vi "Pulse Measurements 1 chan (obs).vi"(6 "percent level settings":T2={"method"=enum."auto select", "histogram size"=256, "histogram method"=enum."mode", "reserved"=1.0} {"reserved" format="%0.2f"}, 7 "pulse number (1)":i32=1 min=1, 8 "error in (no error)":errorcluster, 9 "reference levels":T3={"high ref level"=90.0, "mid ref level"=50.0, "low ref level"=10.0, "ref units"=1} {"ref units" items=["absolute", "percent"]; "high ref level" format="%0.2f"; "low ref level" format="%0.2f"; "mid ref level" format="%0.2f"}, 10 "polarity (high)":u16(ring)=1 items=["low pulse", "high pulse"], 11 "signal in":waveform(dbl)={"t0"=timestamp(0 s since 1904-01-01), "dt"=0.0, "Y"=[]}) -> (0 "error out":errorcluster, 1 "duty cycle":dbl format="%.2g", 2 "pulse duration":dbl format="%.2g", 3 "period":dbl format="%.2g", 4 "measurement info":T1 {"ref levels"."ref units" items=["absolute", "relative"]; "ref levels"."high ref level" format="%.2p"; "ref levels"."low ref level" format="%.2p"; "ref levels"."mid ref level" format="%.2p"; "pulse center" format="%.2p"})   [LabVIEW 2020, in "NI_MAPro.lvlib"]
uses:
  NI_MAPro.lvlib
  <resource>/lvanlys.dll
  NI_MABase.lvlib
panel:
  # "This VI is obsolete !!!\nYou should replace this VI in your diagram with the Pulse Measurements VI."
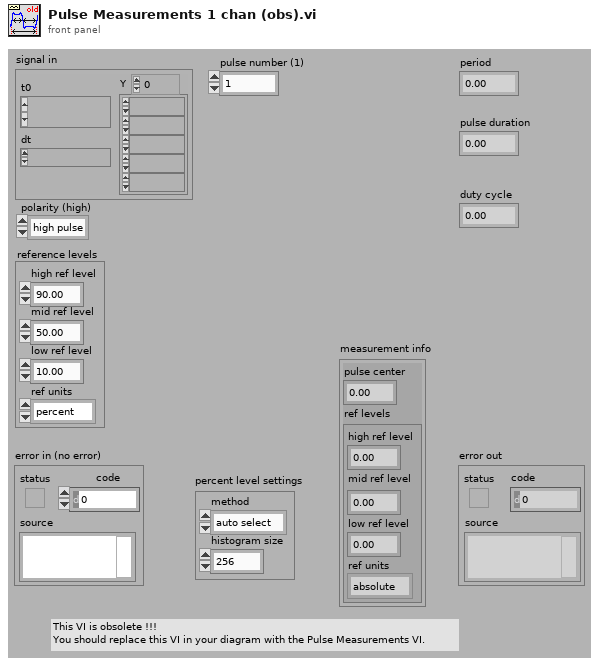
[diagram p1: front panel]
types:
  T1 = cluster{"pulse center":dbl, "ref levels":cluster{"high ref level":dbl, "mid ref level":dbl, "low ref level":dbl, "ref units":u16}}
  T2 = cluster{"method":enum32{"histogram", "peak", "auto select"}, "histogram size":i32, "histogram method":enum16{"mode"}, "reserved":dbl}
  T3 = cluster{"high ref level":dbl, "mid ref level":dbl, "low ref level":dbl, "ref units":u16}
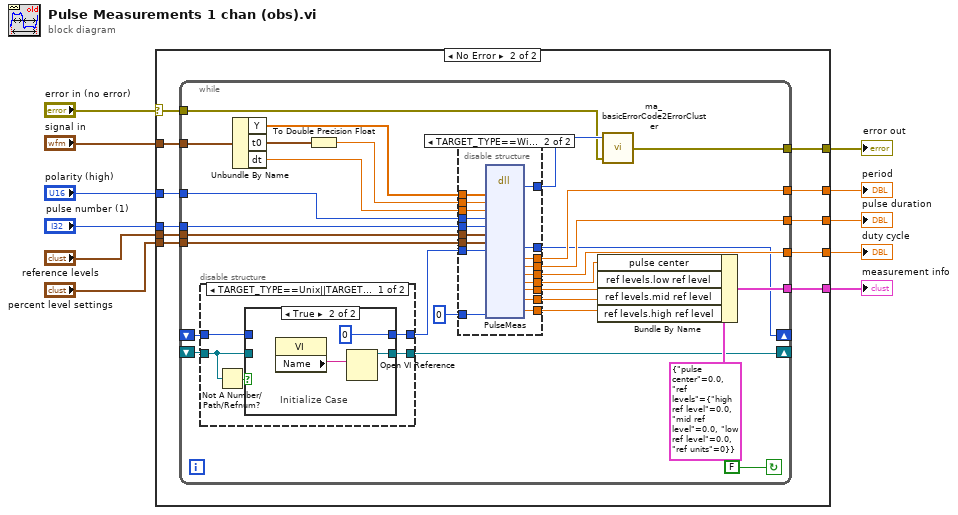
[diagram p0: block diagram]
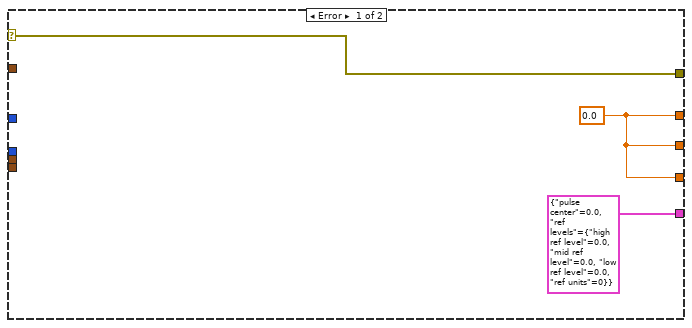
[diagram p2: hidden frame]
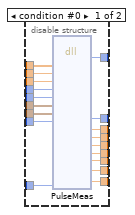
[diagram p3: hidden frame]
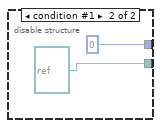
[diagram p5: hidden frame]
diagram:
  n1 = case shown="No Error" "error in (no error)" {
    selector: "error in (no error)" -> [w14 w24]
    tunnel: "polarity (high)" -> [_ w19]
    tunnel: "reference levels" -> [_ w21]
    tunnel: "percent level settings" -> [_ w22]
    tunnel: "pulse number (1)" -> [_ w20]
    tunnel: "signal in" -> [_ w25]
    tunnel: [w14 w15] -> w5
    tunnel: [w13 w16] -> w4
    tunnel: [w13 w17] -> w3
    tunnel: [w13 w18] -> w2
    tunnel: [T1 {"pulse center"=0.0, "ref levels"={"high ref level"=0.0, "mid ref level"=0.0, "low ref level"=0.0, "ref units"=0}} ("measurement info") w23] -> w1
    frame Error {
      w13 = 0.0 ("result")
    }
    frame No Error {
      n2 = while {
        tunnel: w25 -> [w53]
        tunnel: w24 -> [w27]
        tunnel: [w50] -> w23
        tunnel: w22 -> [w49]
        tunnel: w21 -> [w48]
        tunnel: w20 -> [w47]
        tunnel: w19 -> [w46]
        tunnel: [w37] -> w18
        tunnel: [w36] -> w17
        tunnel: [w35] -> w16
        shift-right: [w34] -> _
        shift-left: _ -> [w33]
        shift-right: [w30] -> _
        shift-left: _ -> [w32]
        tunnel: [w26] -> w15
        stop <- FALSE continue-if-true
        n3 = disable-structure shown="TARGET_TYPE==Unix||TARGET_TYPE==Mac||TARGET_TYPE==RT||TARGET_TYPE==Windows, Default" {
          disable-tunnel: w32 -> [w92 _]
          disable-tunnel: [w93 refnum<vi> refnum ("VI Refnum")] -> w30
          disable-tunnel: w33 -> [w91 _]
          disable-tunnel: [w90 0 ("t")] -> w31
          frame condition #0 (active) {
            n4 = Not A Number/Path/Refnum?(number/path/refnum=w92) -> (NaN/Path/Refnum?=w94:bool)
            n5 = case shown="True" w94 {
              tunnel: [w96 w98] -> w93
              tunnel: w92 -> [w96 _]
              tunnel: w91 -> [w95 _]
              tunnel: [w95 0 ("error")] -> w90
              frame False {
              }
              frame True {
                # "Initialize Case"
                n6 = property class="VI"() -> ("Name"=w97:string)  [unwired: 2 in, 2 out]
                n7 = Open VI Reference(vi path=w97) -> (vi reference=w98:refnum<vi>)  [unwired: 1 in, 5 out]
              }
            }
          }
          frame condition #1 {
          }
        }
        n8 = Unbundle By Name(w53) -> ("Y"=w52:dbl[], "t0"=w45:timestamp, "dt"=w43:dbl)
        n9 = To Double Precision Float(number=w45) -> (double precision float=w44:dbl)
        n10 = disable-structure shown="TARGET_TYPE==Windows||TARGET_TYPE==Mac||TARGET_TYPE==Unix||TARGET_BITNESS==64" {
          disable-tunnel: w52 -> [w71 w89]
          disable-tunnel: [w70 w88] -> w28
          disable-tunnel: w49 -> [w69 w87]
          disable-tunnel: w48 -> [w68 w86]
          disable-tunnel: w47 -> [w67 w85]
          disable-tunnel: w46 -> [w66 w84]
          disable-tunnel: w44 -> [w65 w83]
          disable-tunnel: w43 -> [w64 w82]
          disable-tunnel: [w63 w81] -> w41
          disable-tunnel: [w62 w80] -> w40
          disable-tunnel: [w61 w79] -> w39
          disable-tunnel: [w60 w78] -> w38
          disable-tunnel: [w59 w77] -> w37
          disable-tunnel: [w58 w76] -> w36
          disable-tunnel: [w57 w75] -> w35
          disable-tunnel: [w56 w74] -> w34
          disable-tunnel: w31 -> [w55 w73]
          disable-tunnel: 0 ("newAlgorithm") -> [w54 w72]
          frame condition #0 {
            n11 = dll-call lib="C:/Program Files (x86)/National Instruments/LabVIEW 2020/resource/lvanlys.*" fn="PulseMeas"("xH"=w71, "Xo"=w65, "dx"=w64, "polarity"=w66, "pulseNum"=w67, "refLevel"=w68, "percentLevel"=w69, "work"=w55, "newAlgorithm"=w54) -> ("return type"=w70:i32, "work"=w56:i32, "period"=w57:dbl, "pulseDuration"=w58:dbl, "dutyCycle"=w59:dbl, "pulseCenter"=w60:dbl, "lowRefLevel"=w61:dbl, "midRefLevel"=w62:dbl, "highRefLevel"=w63:dbl)  [unwired: 18 in, 2 out]
          }
          frame condition #1 (active) {
            n12 = dll-call lib="C:/Program Files (x86)/National Instruments/LabVIEW 2020/resource/lvanlys.dll" fn="PulseMeas"("xH"=w89, "Xo"=w83, "dx"=w82, "polarity"=w84, "pulseNum"=w85, "refLevel"=w86, "percentLevel"=w87, "work"=w73, "newAlgorithm"=w72) -> ("return type"=w88:i32, "work"=w74:i64, "period"=w75:dbl, "pulseDuration"=w76:dbl, "dutyCycle"=w77:dbl, "pulseCenter"=w78:dbl, "lowRefLevel"=w79:dbl, "midRefLevel"=w80:dbl, "highRefLevel"=w81:dbl)  [unwired: 9 in, 11 out]
          }
        }
        n13 = Bundle By Name(cluster=T1 {"pulse center"=0.0, "ref levels"={"high ref level"=0.0, "mid ref level"=0.0, "low ref level"=0.0, "ref units"=0}} ("measurement info"), "pulse center"=w38, "ref levels.low ref level"=w39, "ref levels.mid ref level"=w40, "ref levels.high ref level"=w41) -> (w50:T1)
        n14 = call "ma_basicErrorCode2ErrorCluster.vi"("error in (no error)"=w27, "Error Code"=w28) -> ("error out"=w26:errorcluster)  [unwired: 1 in]
      }
    }
  }
  "period" <- w4
  "pulse duration" <- w3
  "duty cycle" <- w2
  "error out" <- w5
  "measurement info" <- w1
